vi "Is Allowed Path.vi"(10 "Data Cluster in":T1, 11 "Path":path) -> (3 "Forbidden":bool)   [LabVIEW 2025, in "Scripting Server.lvlib"]
uses:
  Scripting Server.lvlib
  Module Data--cluster.ctl
  Config Data.ctl
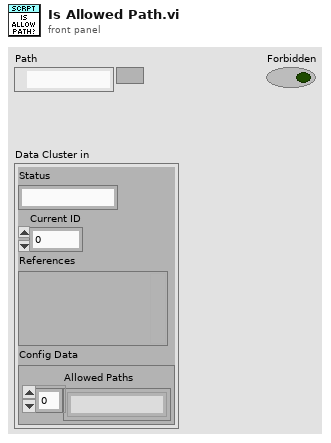
[diagram p1: front panel]
types:
  T1 = typedef "Scripting Server.lvlib/Module Data--cluster.ctl" = cluster{"Status":string, "Current ID":i32, "References":variant, "Config Data":T2}
  T2 = typedef "Scripting Server.lvlib/Config Data.ctl" = cluster{"Allowed Paths":string[]}
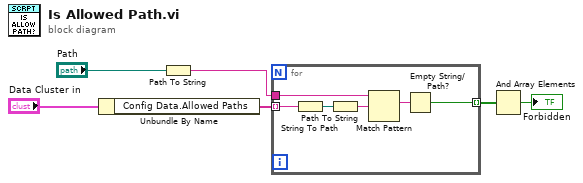
[diagram p0: block diagram]
diagram:
  n1 = Unbundle By Name("Data Cluster in") -> ("Config Data.Allowed Paths"=w6:string[])
  n2 = Path To String(path="Path") -> (string=w2:string)
  n3 = for {
    tunnel: w2 -> [w12]
    tunnel: w6 -> [w8] mode=indexing
    tunnel: [w7] -> w4 mode=indexing
    n4 = String To Path(string=w8) -> (path=w11:path)
    n5 = Path To String(path=w11) -> (string=w10:string)
    n6 = Match Pattern(string=w12, regular expression=w10) -> (match substring=w9:string)  [unwired: 1 in, 3 out]
    n7 = Empty String/Path?(string/path=w9) -> (empty?=w7:bool)
  }
  n8 = And Array Elements(Boolean array=w4) -> (logical AND=→"Forbidden":bool)
